vi "Ball Balancing Table.vi"() -> ()   [LabVIEW 2015]
uses:
  <vilib>/Instr/_visa.llb/Select Event Type.ctl
  <vilib>/FPGAPlugInAG/myRIO-1900/niLvFpga_Open_myRIO-1900.vi
  <vilib>/rvi/interface/common/dynamic/niFpgaDynamicAddResources.vi
  <vilib>/Utility/error.llb/Error Cluster From Error Code.vi
  <vilib>/rvi/errors/niLvFpgaAdjustHostInterfaceError.vi
  <vilib>/FPGAPlugInAG/Dynamic/niLvFpga_Close_Dynamic.vi
  <vilib>/rvi/interface/nirviOpenFPGA/nirviOpenFPGA.xnode
  FPGA Bitfiles/PSM-BallBalancin_FPGATarget_ServoPWMFPGA_nKW44KodaDg.lvbitx
  <vilib>/rvi/interface/nirviReadWriteControl/nirviReadWriteControl.xnode
  <vilib>/rvi/interface/nirviCloseFPGA/nirviCloseFPGA.xnode
  NiFpgaLv.dll
  <vilib>/rvi/interface/Simulation/niFpgaSimulationCallBeginRW.vi
panel:
  in  "Stop":bool
  in  "Play":bool
  in  "PID Y":cluster{"Kp":dbl, "Ki":dbl, "Kd":dbl}
  in  "PID X":cluster{"Kp":dbl, "Ki":dbl, "Kd":dbl}
  out "Y Pixel":u32
  out "X Pixel":u32
  in  "Pattern Menu":enum32{"Point", "Circle", "Lemniscate"}(tab)
  in  "Set Point":cluster{"SetPoint X":dbl, "SetPoint Y":dbl}
  out "Actual Point":cluster{"X Pixel":u32, "Y Pixel":u32}
  in  "Circle Radius (Pixels)":dbl
  in  "Lemniscate Radius (Pixels)":dbl
  out "Error Graph X and Y":cluster{dbl, dbl}(graph)
  out "Measured Y":dbl
  out "Measured X":dbl
  out "Desired Point":cluster{"Desired X":dbl, "Desired Y":dbl}
  out "FPGA VI Reference Out":refnum<k20>
  out "BBT TOUCHSCREEN VISUALIZATION":picture
  # "Ball Balancing Table - BBT"
  # "PID Setting and Controls"
  # "Untuk mendapatkan hasil yang stabil nilai Kp dan Kd\nberturut-turut diisi dengan nilai 0,03 dan 0,01 pada \nmasing-masing axis."
  # "Untuk mendapatkan titik tengah \ndari table isi nilai set-point X dan Y\ndengan nilai 850 pixels"
  # "Input dapat diisi pada rentang \n100-600 pixels untuk mendapatkan \npergerakan pola yang jelas"
  # "Input dapat diisi pada rentang \n100-500 pixels untuk mendapatkan \npergerakan pola yang jelas"
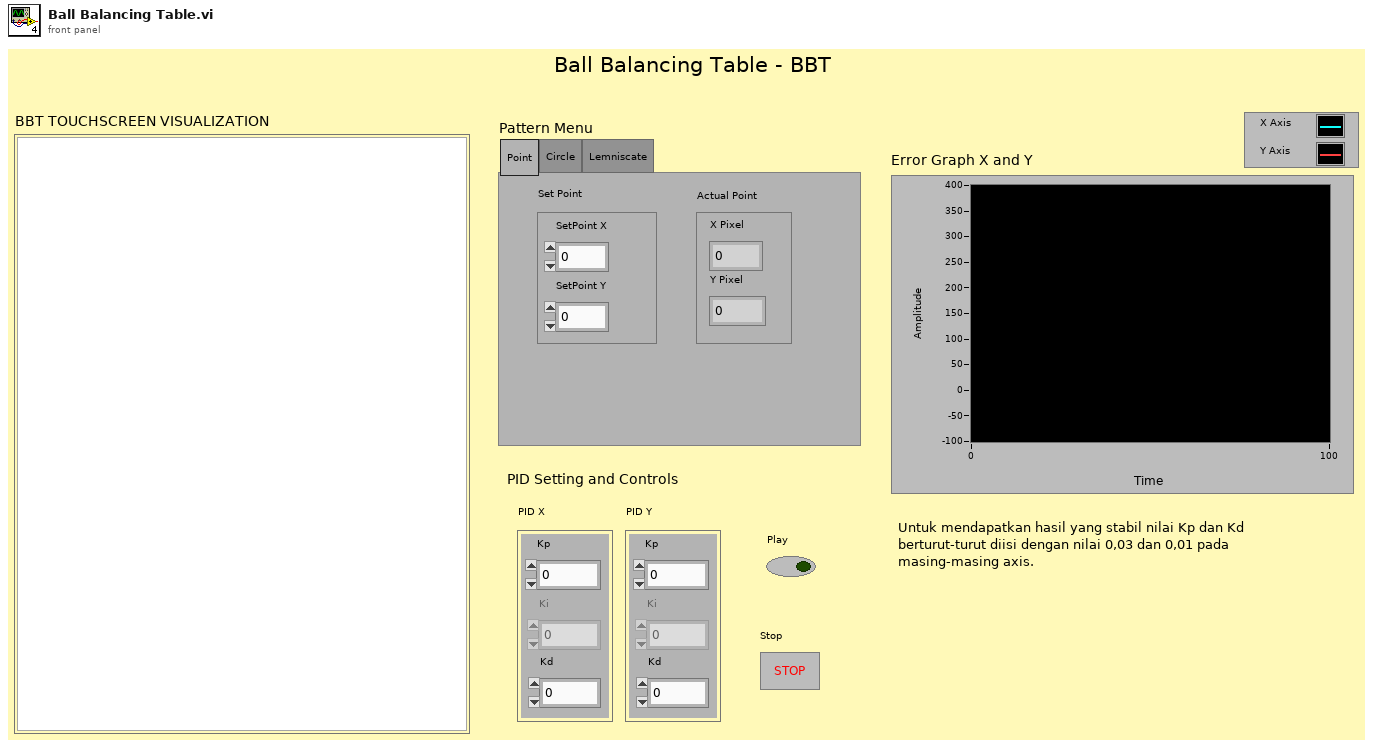
[diagram p1: front panel]
types:
  T1 = typedef "Select Event Type.ctl" = u32
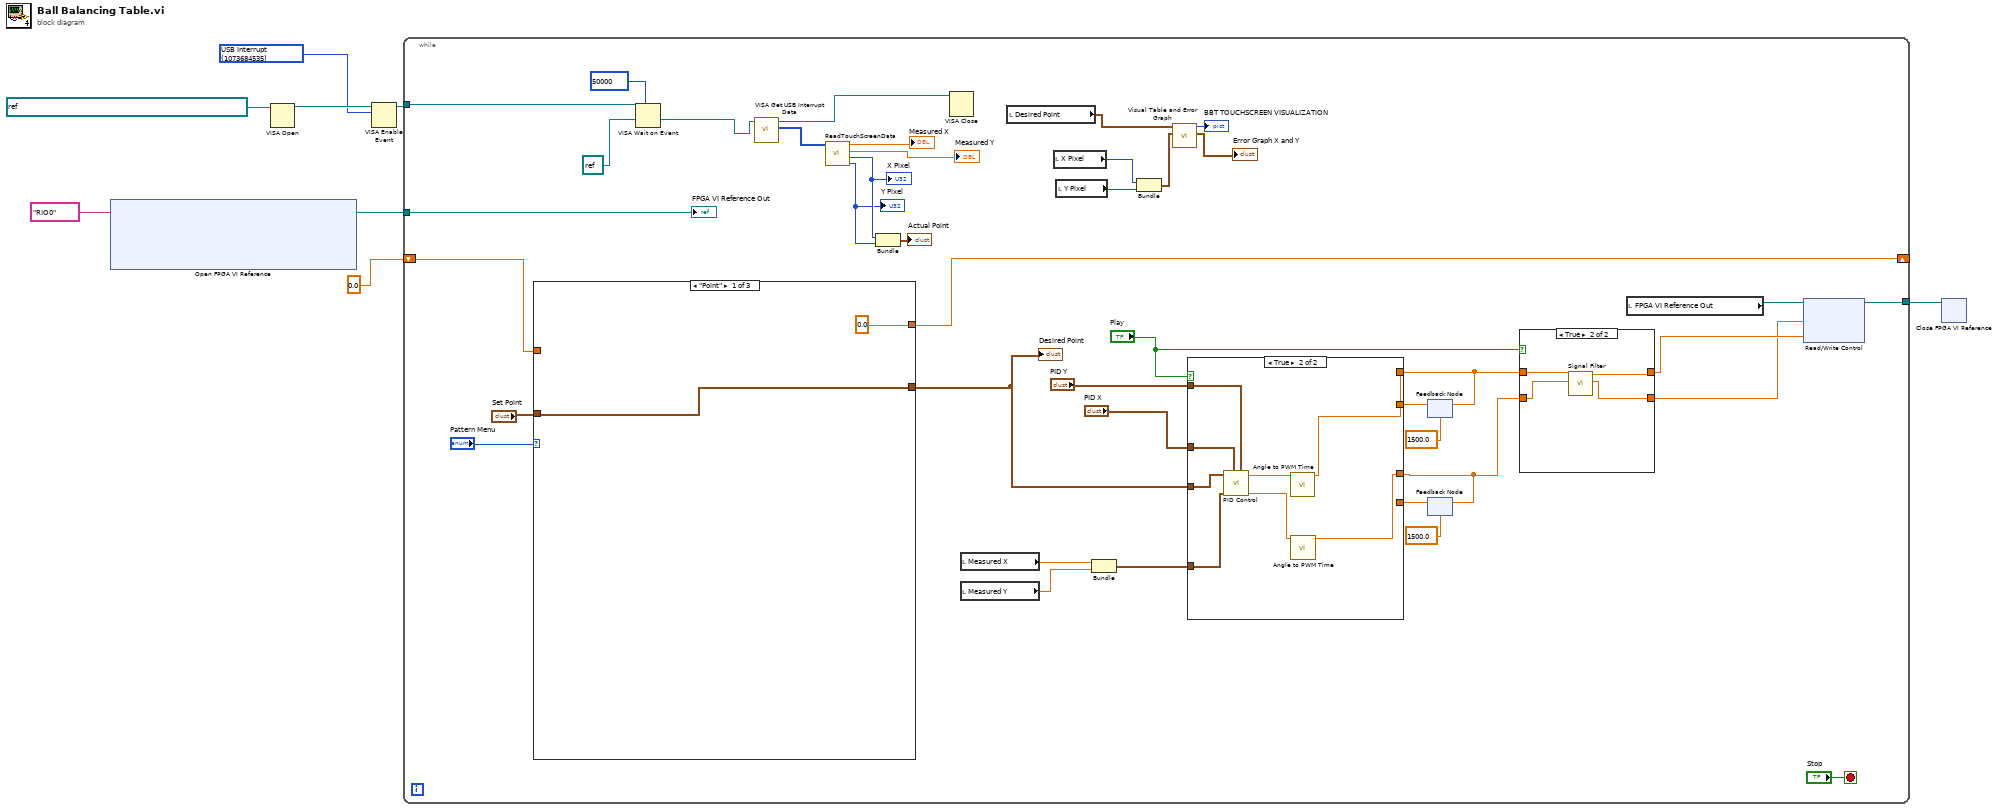
[diagram p0: block diagram]
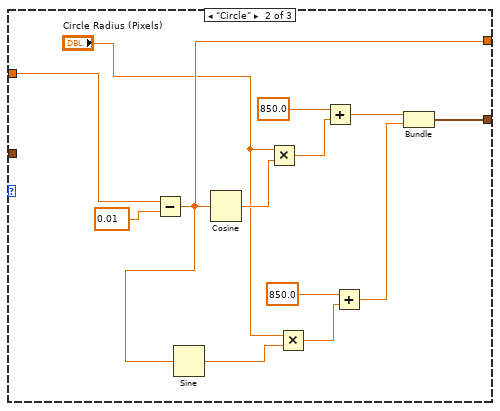
[diagram p4: hidden frame]
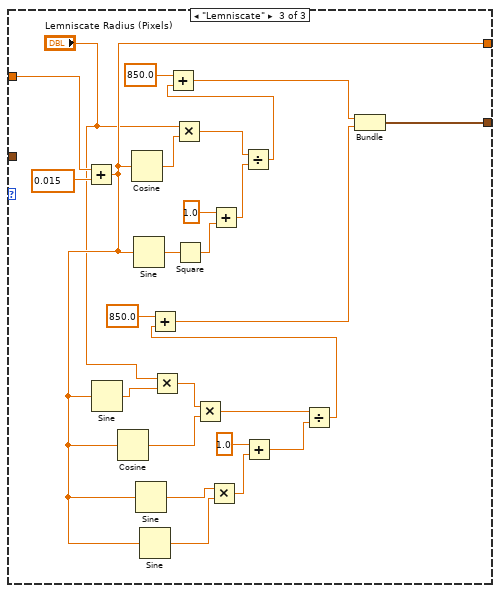
[diagram p5: hidden frame]
diagram:
  w7 = T1 1073684535 items=["Service Request"=1073684491, "Trigger"=3221168138, "Clear"=1073684493, "VXI Signal"=1073684512, "VXI/VME Interrupt"=3221168161, "VXI/VME Sysfail"=1073684509, "VXI/VME Sysreset"=1073684510, "GPIB CIC"=1073684498, "GPIB Talk"=1073684499, "GPIB Listen"=1073684500, "PXI Interrupt"=1073684514, "Serial Break"=1073684515, "Serial TermChar"=1073684516, "Serial CTS"=1073684521, "Serial DSR"=1073684522, "Serial DCD"=1073684524, "Serial RI"=1073684526, "Serial Character"=1073684533, "USB Interrupt"=1073684535, "All Enabled"=1073709055] ("Event Type")
  n1 = xnode "Open FPGA VI Reference"("resource name"=tag "RIO0") -> ("FPGA VI Reference Out"=w4:refnum<k20>)  [unwired: 1 in, 1 out]
  n2 = VISA Open(VISA resource name=refnum<visa-resource-name> "USB0::0x0EEF::0x0001::NI-VISA-1002::RAW") -> (VISA resource name=w8:refnum<visa-resource-name>)  [unwired: 4 in, 1 out]
  n3 = VISA Enable Event(10:w7, 11:w8) -> (3:w6:refnum<visa-resource-name>)  [unwired: 2 in, 1 out]
  n4 = while {
    tunnel: w6 -> [w40]
    tunnel: w4 -> [w36]
    tunnel: [w37] -> w3
    shift-right: [w14] -> _
    shift-left: 0.0 -> [w13]
    stop <- "Stop" stop-if-true
    n5 = case shown="\"Point\"" "Pattern Menu" {
      tunnel: "Set Point" -> [w66 _ _]
      tunnel: [w66 w70 w81] -> w23
      tunnel: w13 -> [_ w76 w96]
      tunnel: [0.0 w68 w84] -> w14
      frame "Point" {
      }
      frame "Circle" {
        n6 = Subtract(x=w76, y=0.01) -> (x-y=w68:dbl)
        n7 = Sine(x=w68) -> (sin(x)=w73:dbl)
        n8 = Cosine(x=w68) -> (cos(x)=w78:dbl)
        n9 = Multiply(x="Circle Radius (Pixels)", y=w78) -> (x*y=w77:dbl)
        n10 = Multiply(x="Circle Radius (Pixels)", y=w73) -> (x*y=w74:dbl)
        n11 = Add(x=850.0, y=w77) -> (x+y=w72:dbl)
        n12 = Add(x=850.0, y=w74) -> (x+y=w71:dbl)
        n13 = Bundle(w72, w71) -> (w70:cluster{dbl, dbl})  [unwired: 1 in]
      }
      frame "Lemniscate" {
        n14 = Add(x=w96, y=0.015) -> (x+y=w84:dbl)
        n15 = Sine(x=w84) -> (sin(x)=w94:dbl)
        n16 = Cosine(x=w84) -> (cos(x)=w92:dbl)
        n17 = Cosine(x=w84) -> (cos(x)=w104:dbl)
        n18 = Sine(x=w84) -> (sin(x)=w102:dbl)
        n19 = Sine(x=w84) -> (sin(x)=w91:dbl)
        n20 = Sine(x=w84) -> (sin(x)=w90:dbl)
        n21 = Multiply(x="Lemniscate Radius (Pixels)", y=w94) -> (x*y=w93:dbl)
        n22 = Multiply(x="Lemniscate Radius (Pixels)", y=w104) -> (x*y=w100:dbl)
        n23 = Square(x=w102) -> (x^2=w101:dbl)
        n24 = Multiply(x=w93, y=w92) -> (x*y=w87:dbl)
        n25 = Multiply(x=w91, y=w90) -> (x*y=w88:dbl)
        n26 = Add(x=1.0, y=w101) -> (x+y=w99:dbl)
        n27 = Divide(x=w100, y=w99) -> (x/y=w98:dbl)
        n28 = Add(x=850.0, y=w98) -> (x+y=w83:dbl)
        n29 = Add(x=1.0, y=w88) -> (x+y=w86:dbl)
        n30 = Divide(x=w87, y=w86) -> (x/y=w85:dbl)
        n31 = Add(x=850.0, y=w85) -> (x+y=w82:dbl)
        n32 = Bundle(w83, w82) -> (w81:cluster{dbl, dbl})  [unwired: 1 in]
      }
    }
    "Desired Point" <- w23
    n33 = VISA Wait on Event(7:u32 50000 ("timeout (0)"), 9:refnum<visa-resource-name> refnum ("event class (Generic Event)"), 11:w40) -> (1:w41:refnum<visa-resource-name>)  [unwired: 2 in, 3 out]
    n34 = call <vilib>:"VISA Get USB Interrupt Data.vi"("VISA USB Intr Event"=w41) -> ("data buffer"=w39:u8[], "VISA USB Intr Event out"=w26:refnum<visa-resource-name>)  [unwired: 8 in, 1 out]
    n35 = call "ReadTouchScreenData.vi"("Interrupt data"=w39) -> ("Y Pixel"=w10:u32, "X Pixel"=w11:u32, "Measured Y"=→"Measured Y":dbl, "Measured X"=→"Measured X":dbl)  [unwired: 6 in]
    "Y Pixel" <- w10
    "X Pixel" <- w11
    n36 = Bundle("X Pixel"=w11, "Y Pixel"=w10) -> (→"Actual Point":cluster{"X Pixel":u32, "Y Pixel":u32})  [unwired: 1 in]
    n37 = VISA Close(VISA resource name=w26) -> ()  [unwired: 1 in, 1 out]
    n38 = local read "Measured X"() -> (w22:dbl)
    n39 = local read "Measured Y"() -> (w21:dbl)
    n40 = local read "Desired Point"() -> (w34:cluster{"Desired X":dbl, "Desired Y":dbl})
    n41 = local read "X Pixel"() -> (w47:u32)
    n42 = local read "Y Pixel"() -> (w46:u32)
    n43 = Bundle("Measured X"=w22, "Measured Y"=w21) -> (w20:cluster{"Measured X":dbl, "Measured Y":dbl})  [unwired: 1 in]
    n44 = Bundle("X Pixel"=w47, "Y Pixel"=w46) -> (w45:cluster{"X Pixel":u32, "Y Pixel":u32})  [unwired: 1 in]
    n45 = call "Visual Table and Error Graph.vi"("Measured Point"=w45, "Set Point"=w34) -> ("Error Graph"=→"Error Graph X and Y":cluster{dbl, dbl}, "new picture"=→"BBT TOUCHSCREEN VISUALIZATION":picture)  [unwired: 8 in]
    n46 = feedback #1(1500.0) -> (w32:dbl)
    n47 = feedback #2(1500.0) -> (w30:dbl)
    n48 = case shown="True" "Play" {
      tunnel: w32 -> [w56 _]
      tunnel: [w56 w61] -> w28
      tunnel: [w55 w60] -> w27
      tunnel: w30 -> [w55 _]
      tunnel: w23 -> [_ w64]
      tunnel: w20 -> [_ w63]
      tunnel: "PID Y" -> [_ w59]
      tunnel: "PID X" -> [_ w58]
      frame False {
      }
      frame True {
        n49 = call "PID Control.vi"("Set Point"=w64, "Actual Value"=w63, "PID Gain X"=w58, "PID Gain Y"=w59) -> ("Output PID X"=w62:dbl, "Output PID Y"=w57:dbl)  [unwired: 5 in]
        n50 = call "Angle to PWM Time.vi"("Angle (degrees)"=w62) -> ("PWM value"=w61:dbl)  [unwired: 10 in]
        n51 = call "Angle to PWM Time.vi"("Angle (degrees)"=w57) -> ("PWM value"=w60:dbl)  [unwired: 10 in]
      }
    }
    n52 = feedback-in #1(w28) -> ()
    n53 = feedback-in #2(w27) -> ()
    n54 = case shown="True" "Play" {
      tunnel: w28 -> [w50 w52]
      tunnel: w27 -> [w49 w51]
      tunnel: [w50 w54] -> w19
      tunnel: [w49 w53] -> w18
      frame False {
      }
      frame True {
        n55 = call "Signal Filter.vi"("Y PWM FPGA"=w51, "X PWM FPGA"=w52) -> ("Y PWM Out"=w53:dbl, "X PWM Out"=w54:dbl)  [unwired: 8 in]
      }
    }
    n56 = local read "FPGA VI Reference Out"() -> (w38:refnum<k20>)
    n57 = xnode "Read/Write Control"("FPGA VI Reference In"=w38, "SERVO X"=w18, "SERVO Y"=w19) -> ("FPGA VI Reference Out"=w37:refnum<k20>)  [unwired: 1 in, 1 out]
    "FPGA VI Reference Out" <- w36
  }
  n58 = xnode "Close FPGA VI Reference"("FPGA VI Reference In"=w3) -> ()  [unwired: 1 in, 1 out]
